vi "Step Counter.Step Count Controller.vi"(10 "Step Action":T2=enum."Data +", 11 "Step State":T1) -> (2 "Step":string, 3 "Step State Out":T1, 5 "Cntr":i32)   [LabVIEW 2018]
uses:
  SubVIs/Step Counter.Action.ctl
  Step Counter.State Info.ctl
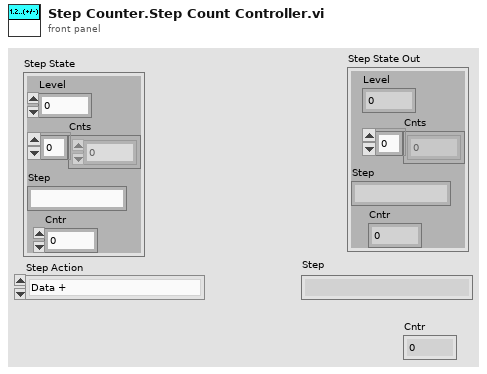
[diagram p1: front panel]
types:
  T1 = typedef "Step Counter.State Info.ctl" = cluster{"Level":i32, "Cnts":i32[], "Step":string, "Cntr":i32}
  T2 = typedef "Step Counter.Action.ctl" = enum16{"Init", "Section Start", "Data +", "Sub Section Start", "Sub Section End", "Get Step"}
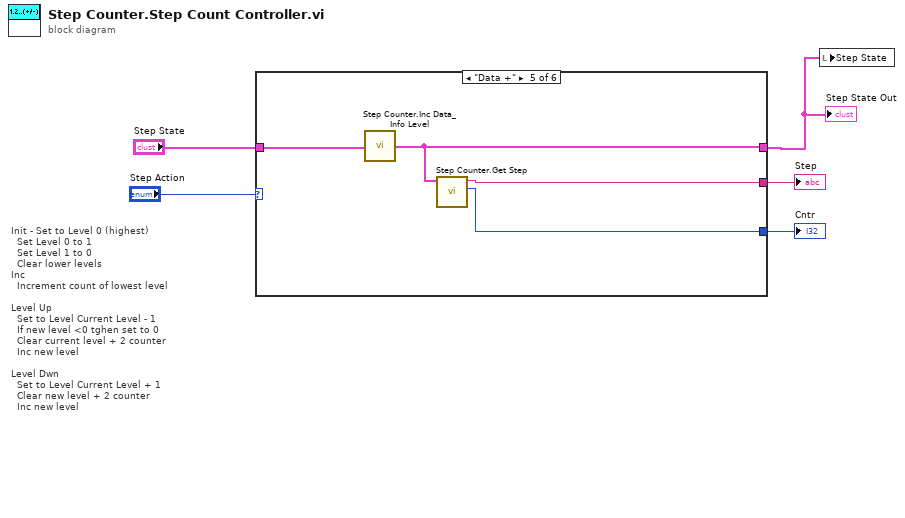
[diagram p0: block diagram]
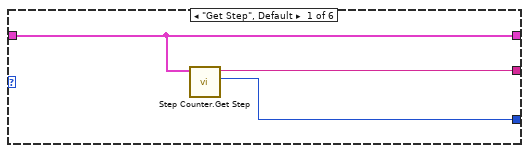
[diagram p2: hidden frame]
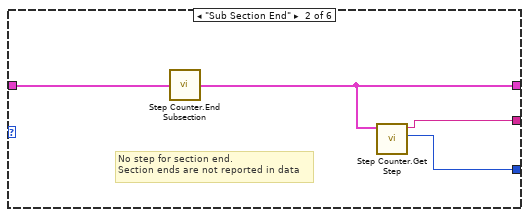
[diagram p3: hidden frame]
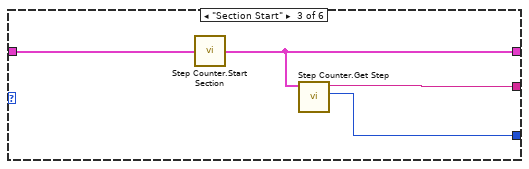
[diagram p4: hidden frame]
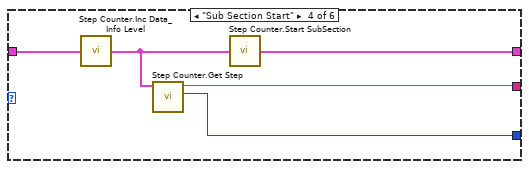
[diagram p5: hidden frame]
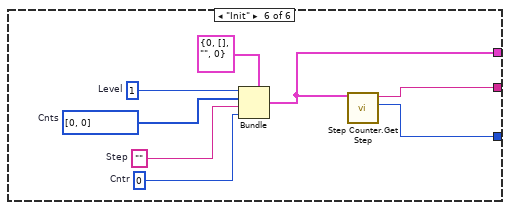
[diagram p6: hidden frame]
diagram:
  # "Init - Set to Level 0 (highest)\n  Set Level 0 to 1\n  Set Level 1 to 0\n  Clear lower levels\nInc\n  Increment count of lowest level\n\nLevel Up\n  Set to Level Current Level - 1\n  If new level <0 tghen set to 0\n  Clear current level + 2 counter\n  Inc new level\n\nLevel Dwn\n  Set to Level Current Level + 1\n  Clear new level + 2 counter\n  Inc new level"
  n1 = case shown="\"Data +\"" "Step Action" {
    tunnel: [w7 w11 w16 w21 w24 w30] -> w3
    tunnel: "Step State" -> [w7 w12 w15 w20 w25 _]
    tunnel: [w8 w10 w14 w18 w23 w29] -> w2
    tunnel: [w6 w9 w13 w17 w22 w26] -> w1
    frame "Get Step", Default {
      n2 = call "Step Counter.Get Step.vi"("Step State"=w7) -> ("Cntr"=w6:i32, "Step"=w8:string)  [unwired: 9 in]
    }
    frame "Sub Section End" {
      # "No step for section end.\nSection ends are not reported in data"
      n3 = call "Step Counter.End Subsection.vi"("Step State"=w12) -> ("Step State Out"=w11:T1)
      n4 = call "Step Counter.Get Step.vi"("Step State"=w11) -> ("Cntr"=w9:i32, "Step"=w10:string)  [unwired: 9 in]
    }
    frame "Section Start" {
      n5 = call "Step Counter.Start Section.vi"("Step State"=w15) -> ("Step State Out"=w16:T1)
      n6 = call "Step Counter.Get Step.vi"("Step State"=w16) -> ("Cntr"=w13:i32, "Step"=w14:string)  [unwired: 9 in]
    }
    frame "Sub Section Start" {
      n7 = call "Step Counter.Inc Data_Info Level.vi"("Step State"=w20) -> ("Step State Out"=w19:T1)
      n8 = call "Step Counter.Get Step.vi"("Step State"=w19) -> ("Cntr"=w17:i32, "Step"=w18:string)  [unwired: 9 in]
      n9 = call "Step Counter.Start SubSection.vi"("Step State"=w19) -> ("Step State Out"=w21:T1)
    }
    frame "Data +" {
      n10 = call "Step Counter.Inc Data_Info Level.vi"("Step State"=w25) -> ("Step State Out"=w24:T1)
      n11 = call "Step Counter.Get Step.vi"("Step State"=w24) -> ("Cntr"=w22:i32, "Step"=w23:string)  [unwired: 9 in]
    }
    frame "Init" {
      w28 = 0  # Cntr
      w31 = ""  # Step
      w32 = i32[] [0, 0]  # Cnts
      w33 = 1  # Level
      n12 = Bundle(cluster=T1 {"Level"=0, "Cnts"=[], "Step"="", "Cntr"=0} ("Step State"), "Level"=w33, "Cnts"=w32, "Step"=w31, "Cntr"=w28) -> (w30:T1)
      n13 = call "Step Counter.Get Step.vi"("Step State"=w30) -> ("Cntr"=w26:i32, "Step"=w29:string)  [unwired: 9 in]
    }
  }
  "Step" <- w2
  "Step State Out" <- w3
  "Cntr" <- w1
  n14 = local write "Step State"(w3) -> ()
